vi "数据查询筛选弹框.vi"(8 "error in (no error)":errorcluster caption="错误输入（无错误）", 9 "是否初始化":enum16{"init", "keep"}(ring), 10 "database":string="database1.mdb", 11 "table":string(combo)="CODMn") -> (0 "error out":errorcluster caption="错误输出", 1 "确定输出":bool, 2 "显示项":string[](array[string]), 3 "condition":string)   [LabVIEW 2016]
uses:
  <vilib>/addons/database/Auxilliary.llb/DB Tools DataTypes.ctl
  <vilib>/picture/picture.llb/imagedata.ctl
  <vilib>/Utility/miscctls.llb/LVPointTypeDef.ctl
  <vilib>/Utility/sysdir.llb/System Directory Type.ctl
  <vilib>/addons/database/Connection.llb/DB Tools Open Connec (String).vi
  <vilib>/addons/database/Connection.llb/Conn Execute.vi
  <vilib>/addons/database/Recordset.llb/Rec Fetch Recordset Data (R).vi
  <vilib>/addons/database/Recordset.llb/Rec Destroy - Connection.vi
  <userlib>/_OpenG.lib/array/array.llb/Remove Duplicates from 1D Array (String)__ogtk.vi
  <vilib>/addons/database/_DB Variant To Data/Database Variant To Data.xnode
  <vilib>/addons/database/NI_Database_API.lvlib
panel:
  in  "背景图像":T1
  in  "实时分钟小时数据":enum32{"实时数据", "分钟数据", "小时数据"}(radio)
  in  "确定":bool
  out "自定义2single":cluster{"起始范围":string, "截止范围":string}
  out "自定义1single":cluster{"起始范围":string, "截止范围":string}
  out "自定义2筛选条件":string[](array[string])
  out "自定义1筛选条件":string[](array[string])
  in  "标签 2":string="从：\n\n\n至："
  in  "自定义数值结束 2":dbl
  in  "自定义数值起始 2":dbl
  in  "自定义结束时间 2":timestamp(xcontrol)
  in  "自定义起始时间 2":timestamp(xcontrol)
  in  "自定义 2":T2 caption="自定义"
  in  "下拉列表":string(xcontrol)
  in  "标签":string="从：\n\n\n至："
  in  "自定义数值结束":dbl
  in  "自定义数值起始":dbl
  in  "自定义结束时间":timestamp(xcontrol)
  in  "自定义起始时间":timestamp(xcontrol)
  in  "自定义":T2
  in  "下拉列表 2":string(xcontrol)
  out "type":T3[](array[typedef])
  out "所有测量模式":string[](array[string])
  out "数组":string[](array[string])
  out "columns":string[](array[string])
  in  "测量模式":T4
  in  "退出":bool
  in  "清空":bool
  in  "时间标识输入1":timestamp(xcontrol)
  in  "时间标识输入2":timestamp(xcontrol)
  # "时间"
  # "从："
  # "至："
  # "测试模式"
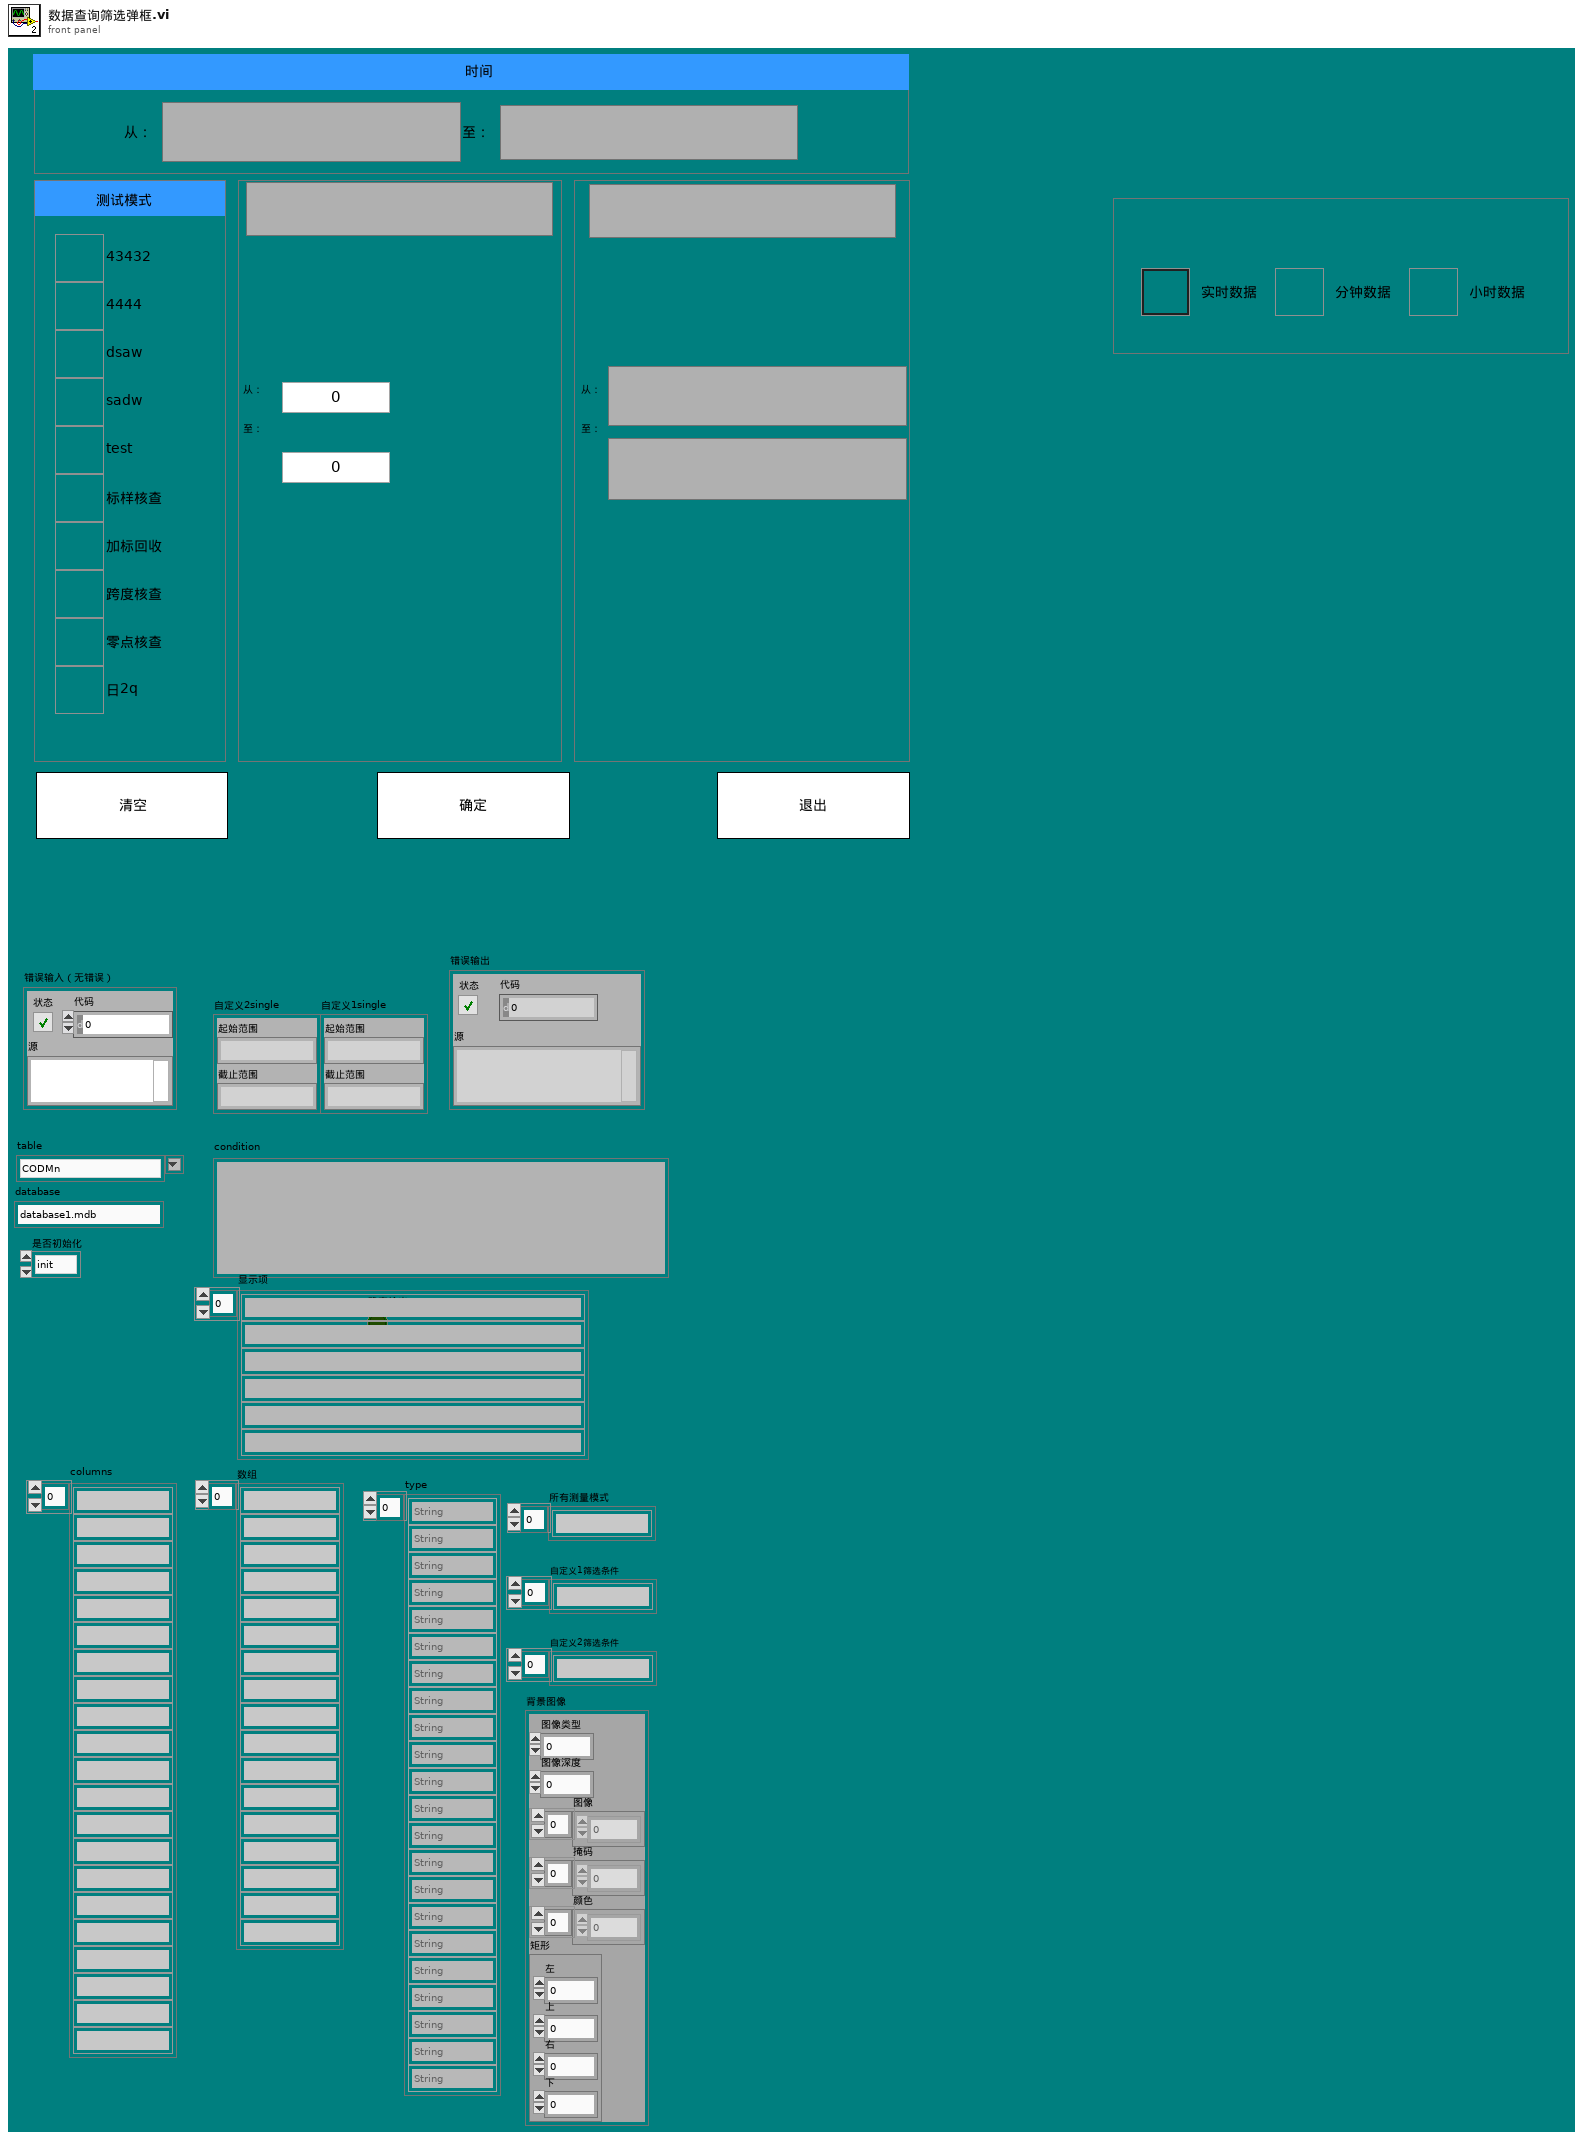
[diagram p1: front panel]
types:
  T1 = typedef "imagedata.ctl" = cluster{"image type":i32, "image depth":i32, "image":u8[], "mask":u8[], "colors":u32[], "Rectangle":cluster{"left":i16, "top":i16, "right":i16, "bottom":i16}}
  T2 = cluster{"DSADSA ":bool, "2":bool, "3":bool, "4":bool, "5":bool, "6":bool, "7":bool, "8":bool, "9":bool, "10":bool}
  T3 = typedef "NI_Database_API.lvlib/DB Tools DataTypes.ctl" = enum16{"String", "Long (I32)", "Single (SGL)", "Double (DBL)", "Date/Time", "Binary"}
  T4 = cluster{"水样测试":bool, "标样核查":bool, "零点核查":bool, "跨度核查":bool, "空白测试":bool, "平行样测试":bool, "加标回收":bool, "空白校准":bool, "标样校准":bool, "初始化清洗":bool}
  T5 = enum8{"Enabled", "Disabled", "Disabled and Grayed Out"}
  T6 = typedef "LVPointTypeDef.ctl" = cluster{"Horizontal":i16, "Vertical":i16}
  T7 = typedef "System Directory Type.ctl" = i32
  T8 = typedef "NI_Database_API.lvlib/Conn ObjectReference.ctl" = refnum<k1>
  T9 = cluster{"name":string, "database data type":T3, "defined size":i32}[]
  T10 = typedef "NI_Database_API.lvlib/Rec ObjectReference.ctl" = refnum<k1>
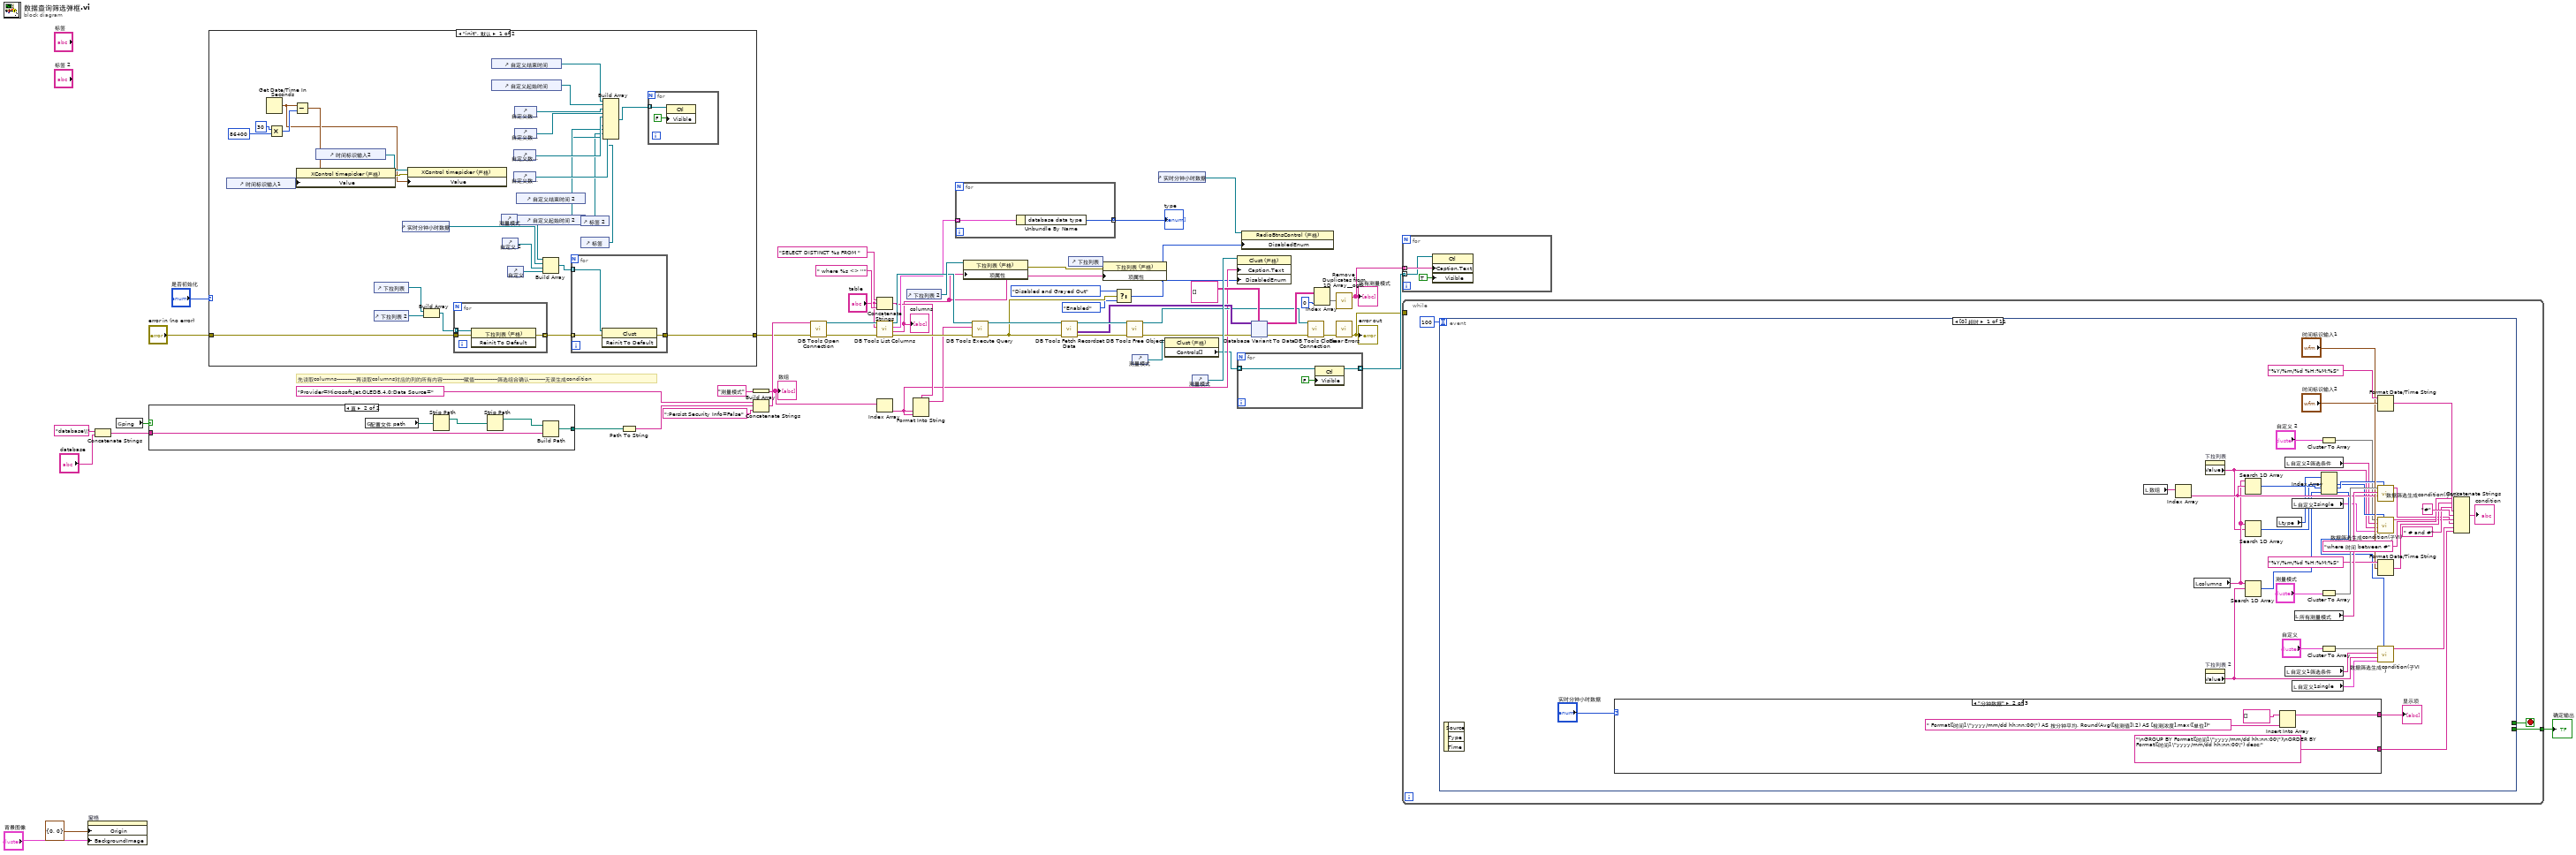
[diagram p0: block diagram]
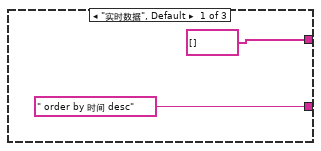
[diagram p3: hidden frame]
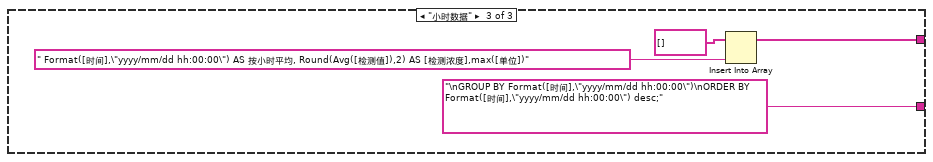
[diagram p4: hidden frame]
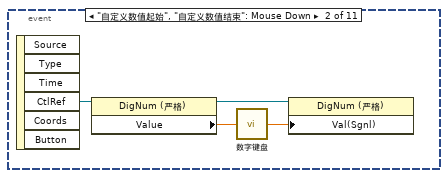
[diagram p5: hidden frame]
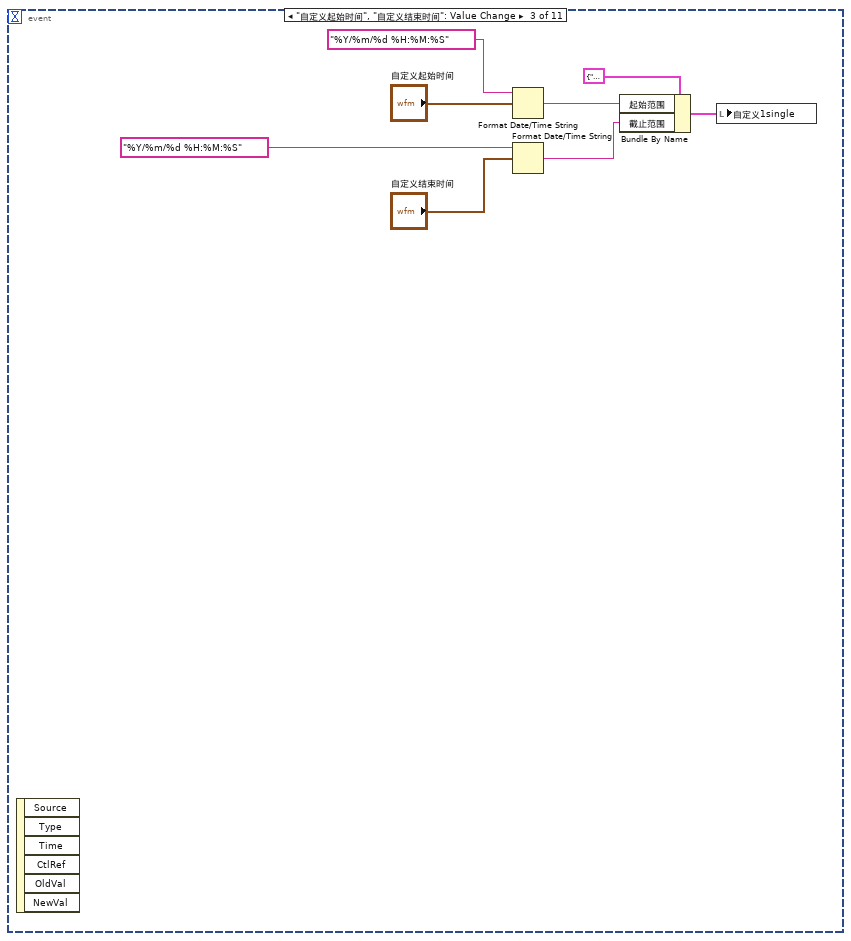
[diagram p6: hidden frame]
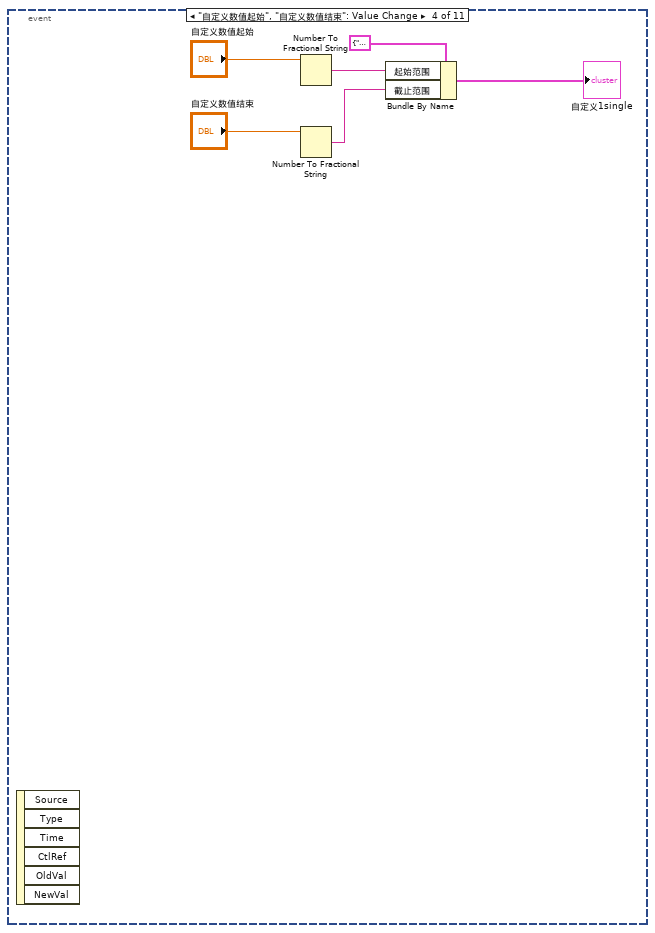
[diagram p7: hidden frame]
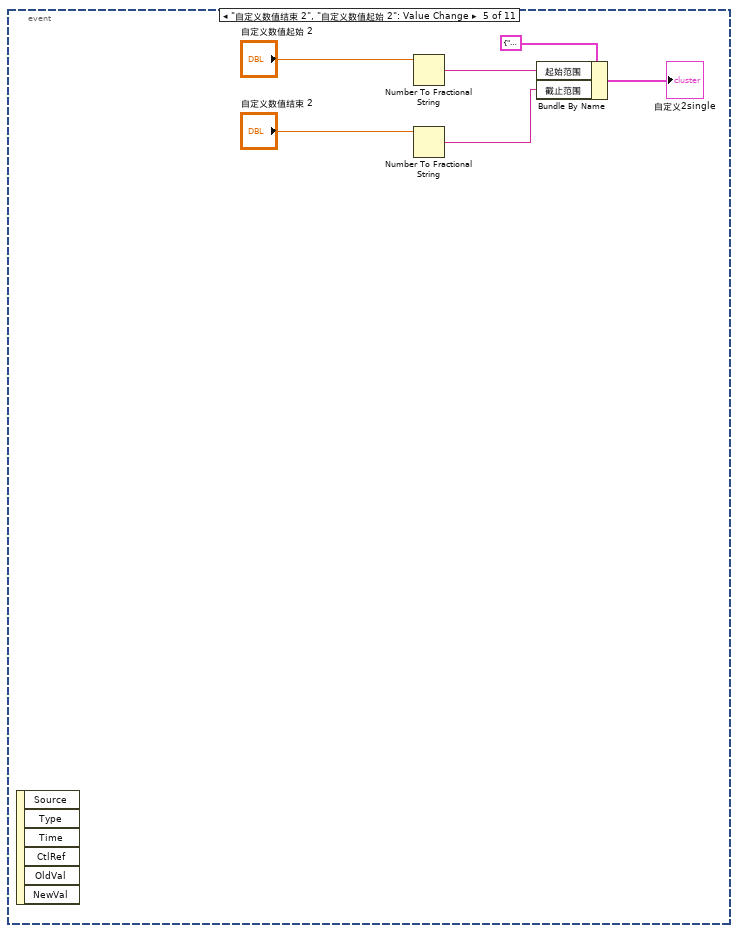
[diagram p8: hidden frame]
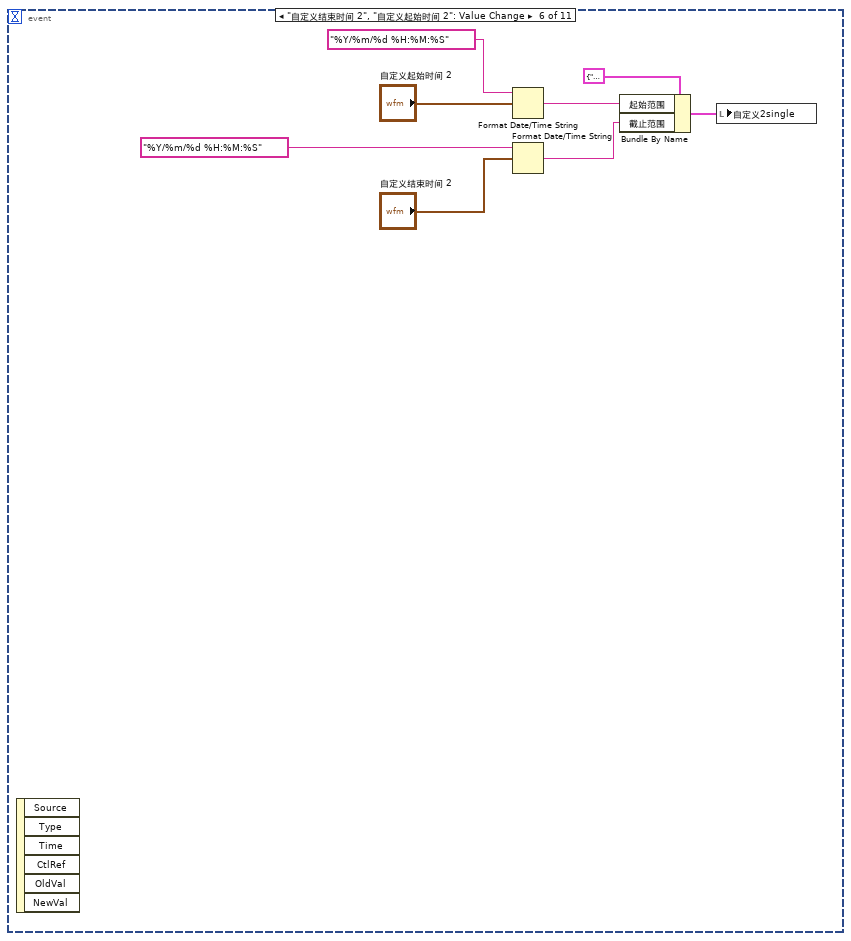
[diagram p9: hidden frame]
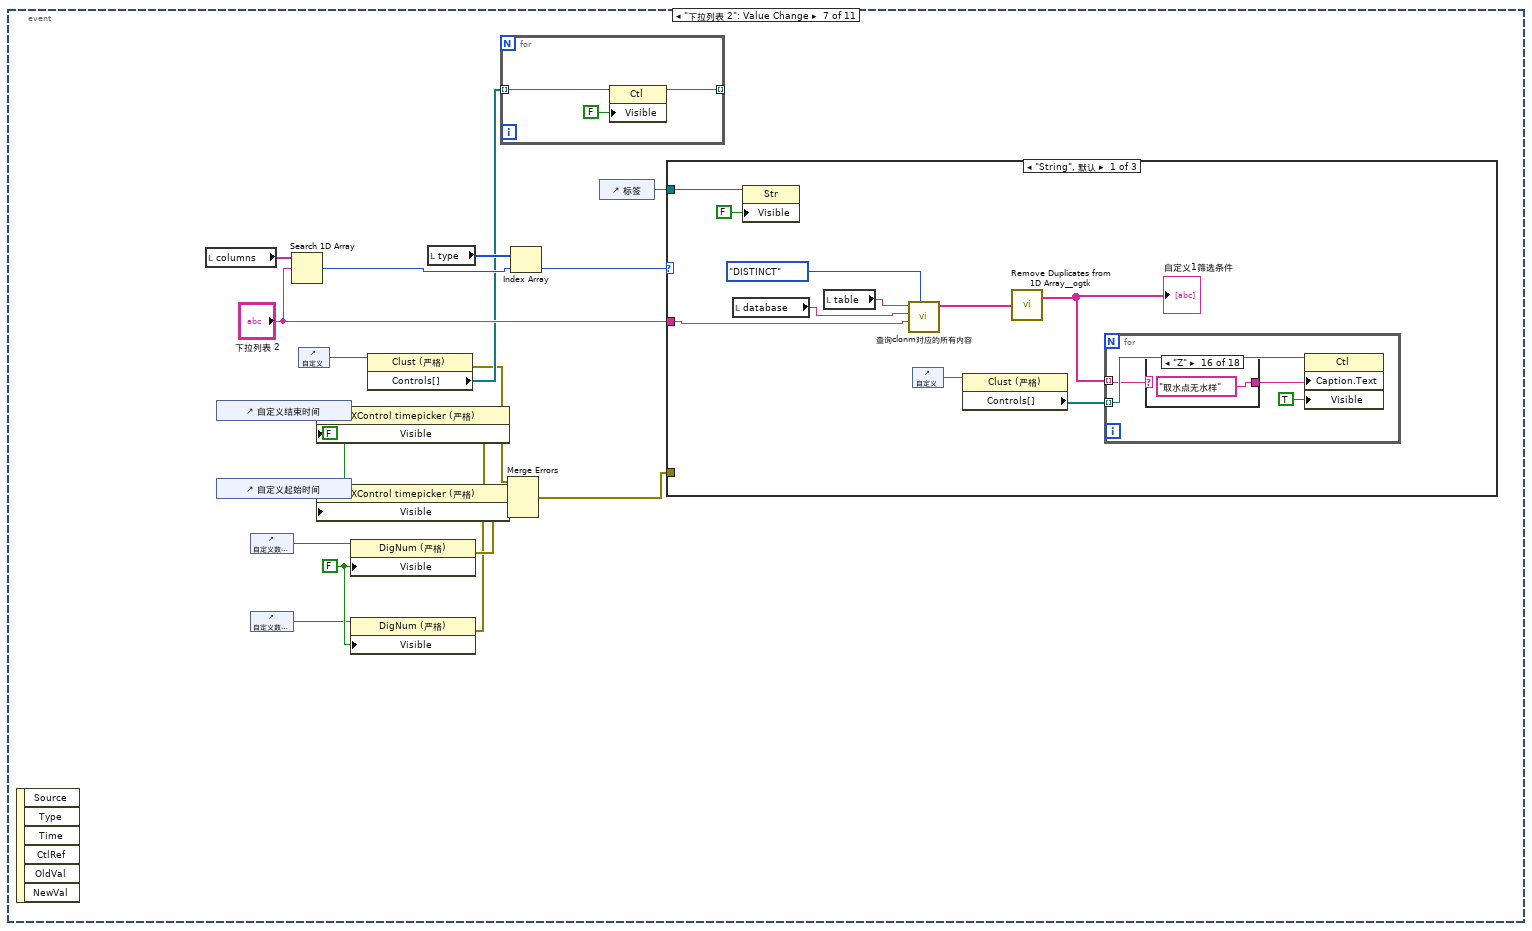
[diagram p10: hidden frame]
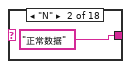
[diagram p12: hidden frame]
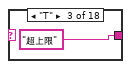
[diagram p13: hidden frame]
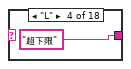
[diagram p14: hidden frame]
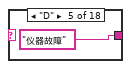
[diagram p15: hidden frame]
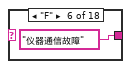
[diagram p16: hidden frame]
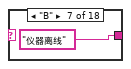
[diagram p17: hidden frame]
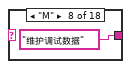
[diagram p18: hidden frame]
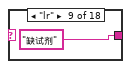
[diagram p19: hidden frame]
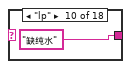
[diagram p20: hidden frame]
diagram:
  # "先读取columns-----------再读取columns对应的列的所有内容------------赋值-------------筛选组合确认---------无误生成condition"
  n1 = property on="窗格" class="Pane"("Origin"=T6 {"Horizontal"=0, "Vertical"=0} ("原点"), "BackgroundImage"="背景图像") -> ()  [unwired: 2 in, 2 out]
  n2 = Concatenate Strings("database\\" ("名称或相对路径"), "database") -> (w48:string)
  n3 = global read "ping全局.vi" "ping"() -> (w49:bool)
  n4 = case shown="真" w49 {
    tunnel: w48 -> [w58 w64]
    tunnel: [w57 w62] -> w47
    frame False {
      w59 = T7 2 items=["用户目录"=0, "用户桌面"=1, "用户文档"=2, "用户应用程序数据"=3, "用户设置"=4, "用户临时目录"=5, "公共文档"=6, "公共应用程序数据"=7, "公共设置"=8, "公共缓存"=13, "系统核心库"=9, "系统安装库"=10, "应用程序文件"=11, "启动盘根目录"=12] ("system directory type")
      n5 = call <vilib>:"Get System Directory.vi"("system directory type"=w59) -> ("system directory"=w60:path)  [unwired: 10 in]
      n6 = Build Path(base path=w60, name or relative path=w58) -> (appended path=w57:path)
    }
    frame True {
      n7 = global read "ping全局.vi" "配置文件 path"() -> (w61:path)
      n8 = Strip Path(path=w61) -> (stripped path=w65:path)  [unwired: 1 out]
      n9 = Strip Path(path=w65) -> (stripped path=w63:path)  [unwired: 1 out]
      n10 = Build Path(base path=w63, name or relative path=w64) -> (appended path=w62:path)
    }
  }
  n11 = case shown="\"init\", 默认" "是否初始化" {
    tunnel: "error in (no error)" -> [w71 w104]
    tunnel: [w90 w104] -> w8
    frame "init", Default {
      n12 = control-ref of="时间标识输入1"() -> (w73:refnum<vi>)
      n13 = Get Date/Time In Seconds() -> (seconds since 1Jan1904=w66:timestamp)
      n14 = Multiply(x=30, y=86400) -> (x*y=w85:i32)
      n15 = Subtract(x=w66, y=w85) -> (x-y=w89:timestamp)
      n16 = property class="XControl timepicker (严格)"(reference=w73, "Value"=w89) -> (error out=w88:errorcluster)  [unwired: 1 in, 1 out]
      n17 = control-ref of="时间标识输入2"() -> (w72:refnum<vi>)
      n18 = control-ref of="下拉列表"() -> (w69:refnum<vi>)
      n19 = control-ref of="下拉列表 2"() -> (w68:refnum<vi>)
      n20 = control-ref of="实时分钟小时数据"() -> (w95:refnum<vi>)
      n21 = property class="XControl timepicker (严格)"(reference=w72, error in=w88, "Value"=w66) -> ()  [unwired: 2 out]
      n22 = Build Array(w69, w68) -> (w67:refnum<vi>[])
      n23 = for {
        tunnel: w71 -> [w98]
        tunnel: [w97] -> w70 mode=indexing
        tunnel: w67 -> [w96] mode=indexing
        n24 = invoke class="下拉列表 (严格)" method="Reinit To Default"(reference=w96, error in=w98) -> (error out=w97:errorcluster)  [unwired: 1 in, 2 out]
      }
      n25 = control-ref of="自定义结束时间"() -> (w84:refnum<vi>)
      n26 = control-ref of="自定义起始时间"() -> (w83:refnum<vi>)
      n27 = control-ref of="测量模式"() -> (w91:refnum<vi>)
      n28 = control-ref of="自定义 2"() -> (w94:refnum<vi>)
      n29 = control-ref of="自定义"() -> (w93:refnum<vi>)
      n30 = control-ref of="自定义数值结束 2"() -> (w80:refnum<vi>)
      n31 = control-ref of="自定义数值起始 2"() -> (w79:refnum<vi>)
      n32 = control-ref of="自定义数值结束"() -> (w82:refnum<vi>)
      n33 = control-ref of="自定义数值起始"() -> (w81:refnum<vi>)
      n34 = control-ref of="自定义结束时间 2"() -> (w77:refnum<vi>)
      n35 = control-ref of="自定义起始时间 2"() -> (w78:refnum<vi>)
      n36 = Build Array(w91, w95, w94, w93) -> (w92:refnum<vi>[])
      n37 = for {
        tunnel: w92 -> [w103] mode=indexing
        tunnel: w70 -> [w102] mode=indexing
        tunnel: [w101] -> w90
        n38 = invoke class="Clust" method="Reinit To Default"(reference=w103, error in=w102) -> (error out=w101:errorcluster)  [unwired: 1 in, 2 out]
      }
      n39 = control-ref of="标签 2"() -> (w74:refnum<vi>)
      n40 = control-ref of="标签"() -> (w75:refnum<vi>)
      n41 = Build Array(w84, w83, w82, w81, w80, w79, w77, w78, w74, w75) -> (w76:refnum<vi>[])
      n42 = for {
        tunnel: w76 -> [w100] mode=indexing
        n43 = property class="Ctl"(reference=w100, "Visible"=FALSE ("可见")) -> ()  [unwired: 1 in, 2 out]
      }
    }
    frame "keep" {
    }
  }
  n44 = Path To String(path=w47) -> (string=w53:string)
  n45 = Build Array("测量模式" ("Element Data")) -> (w11:string[])
  "数组" <- w11
  n46 = Concatenate Strings("Provider=Microsoft.Jet.OLEDB.4.0;Data Source=", w53, ";Persist Security Info=False") -> (w52:string)
  n47 = call-poly <vilib>:"DB Tools Open Connection.vi"("error in (no error)"=w8, "connection information"=w52) -> ("error out"=w45:errorcluster, "connection reference"=w46:T8)  [unwired: 6 in]
  n48 = Concatenate Strings("SELECT DISTINCT %s FROM " ("字符串"), "table", " where %s <> ''" ("字符串")) -> (w22:string)
  n49 = call <vilib>:"DB Tools List Columns.vi"("error in (no error)"=w45, "table"="table", "connection reference"=w46) -> ("error out"=w39:errorcluster, "columns"=w1:string[], "column information"=w26:T9, "connection reference out"=w27:T8)  [unwired: 1 in]
  "columns" <- w1
  n50 = Index Array(array=w11) -> (element=w20:string)  [unwired: 1 in]
  n51 = control-ref of="下拉列表 2"() -> (w28:refnum<vi>)
  n52 = Format Into String(format string=w22, w20, w20) -> (resulting string=w38:string)  [unwired: 2 in, 1 out]
  n53 = for {
    tunnel: w26 -> [w106] mode=indexing
    tunnel: [w105] -> w25 mode=indexing
    n54 = Unbundle By Name(w106) -> ("database data type"=w105:T3)
  }
  "type" <- w25
  n55 = property class="下拉列表 (严格)"(reference=w28, "项属性"=w1) -> (error out=w7:errorcluster)  [unwired: 1 in, 1 out]
  n56 = call-poly <vilib>:"DB Tools Execute Query.vi"("error in (no error)"=w39, "SQL query"=w38, "connection reference"=w27) -> ("error out"=w19:errorcluster, "recordset reference"=w42:T10)  [unwired: 5 in]
  n57 = call-poly <vilib>:"DB Tools Fetch Recordset Data.vi"("error in (no error)"=w19, "recordset reference"=w42) -> ("error out"=w41:errorcluster, "recordset data"=w34:variant[][], "recordset reference out"=w40:T10)  [unwired: 3 in]
  n58 = control-ref of="下拉列表"() -> (w16:refnum<vi>)
  n59 = property class="下拉列表 (严格)"(reference=w16, error in=w7, "项属性"=w1) -> ()  [unwired: 2 out]
  n60 = Select(t=T5."Disabled and Grayed Out" ("禁用"), s=w19, f=T5."Enabled" ("禁用")) -> (s? t:f=w3:T5)
  n61 = call-poly <vilib>:"DB Tools Free Object.vi"("error in (no error)"=w41, "recordset reference"=w40) -> ("error out"=w33:errorcluster, "connection reference"=w32:T8)  [unwired: 8 in]
  n62 = control-ref of="测量模式"() -> (w56:refnum<vi>)
  n63 = control-ref of="实时分钟小时数据"() -> (w4:refnum<vi>)
  n64 = property class="Clust (严格)"(reference=w56) -> ("Controls[]"=w15:refnum<vi>[])  [unwired: 1 in, 2 out]
  n65 = control-ref of="测量模式"() -> (w43:refnum<vi>)
  n66 = property class="Clust (严格)"(reference=w43, "Caption.Text"=w20, "DisabledEnum"=w3) -> ()  [unwired: 1 in, 2 out]
  n67 = for {
    tunnel: w15 -> [w109] mode=indexing
    tunnel: [w107] -> w14 mode=indexing
    n68 = property class="Ctl"(reference=w109, "Visible"=FALSE ("可见")) -> (reference out=w107:refnum<vi>)  [unwired: 1 in, 1 out]
  }
  n69 = property class="RadioBtnsControl (严格)"(reference=w4, "DisabledEnum"=w3) -> ()  [unwired: 1 in, 2 out]
  n70 = xnode "Database Variant To Data"("database variant"=w34, "error in (no error)"=w33, "type"=string[][] []) -> ("data"=w35:string[][], "error out"=w36:errorcluster)
  n71 = call <vilib>:"DB Tools Close Connection.vi"("error in (no error)"=w36, "connection reference"=w32) -> ("error out"=w10:errorcluster)  [unwired: 5 in]
  n72 = Index Array(array=w35, index (col)=0 ("禁用的索引 (列)")) -> (element=w30:string[])  [unwired: 1 in]
  n73 = call-poly <userlib>:"Remove Duplicates from 1D Array__ogtk.vi"("Input Array"=w30) -> ("Output Array"=w13:string[])  [unwired: 1 out]
  "所有测量模式" <- w13
  n74 = call <vilib>:"Clear Errors.vi"("error in (no error)"=w10) -> ("error out"=w5:errorcluster)  [unwired: 5 in, 1 out]
  "error out" <- w5
  n75 = for {
    tunnel: w13 -> [w112] mode=indexing
    tunnel: w14 -> [w110] mode=indexing
    n76 = property class="Ctl"(reference=w110, "Caption.Text"=w112, "Visible"=TRUE ("可见")) -> ()  [unwired: 1 in, 2 out]
  }
  n77 = while {
    tunnel: [w113] -> w12
    tunnel: w5 -> [_]
    stop <- w115 stop-if-true
    n78 = event shown="[0] 超时" {
      selector: _ -> [_ _ _ _ _ _ _ _ _ _ _]
      dyn-events: _ -> [_ _ _ _ _ _ _ _ _ _ _]
      timeout: 100 -> [_ _ _ _ _ _ _ _ _ _ _]
      tunnel: [_ _ _ _ _ _ _ _ _ w395 TRUE] -> w115
      tunnel: [_ _ _ _ _ _ _ _ _ w395 _] -> w113
      event Timeout {
        n79 = event-data() -> ()  [unwired: 1 in, 3 out]
        n80 = case shown="\"分钟数据\"" "实时分钟小时数据" {
          tunnel: [string[] [] ("显示项") w157 w161] -> w116
          tunnel: [" order by 时间 desc" ("字符串") "\nGROUP BY Format([时间],\"yyyy/mm/dd hh:nn:00\")\nORDER BY Format([时间],\"yyyy/mm/dd hh:nn:00\") desc;" ("字符串") "\nGROUP BY Format([时间],\"yyyy/mm/dd hh:00:00\")\nORDER BY Format([时间],\"yyyy/mm/dd hh:00:00\") desc;" ("字符串")] -> w117
          frame "实时数据", Default {
          }
          frame "分钟数据" {
            n81 = Insert Into Array(array=string[] [] ("显示项"), new element=" Format([时间],\"yyyy/mm/dd hh:nn:00\") AS 按分钟平均, Round(Avg([检测值]),2) AS [检测浓度],max([单位])" ("新元素/子数组")) -> (w157:string[])  [unwired: 1 in]
          }
          frame "小时数据" {
            n82 = Insert Into Array(array=string[] [] ("显示项"), new element=" Format([时间],\"yyyy/mm/dd hh:00:00\") AS 按小时平均, Round(Avg([检测值]),2) AS [检测浓度],max([单位])" ("新元素/子数组")) -> (w161:string[])  [unwired: 1 in]
          }
        }
        "显示项" <- w116
        n83 = local read "数组"() -> (w154:string[])
        n84 = Index Array(array=w154) -> (element=w140:string)  [unwired: 1 in]
        n85 = local read "columns"() -> (w134:string[])
        n86 = property on="下拉列表" class="下拉列表 (严格)"() -> ("Value"=w125:string)  [unwired: 2 in, 2 out]
        n87 = property on="下拉列表 2" class="下拉列表 (严格)"() -> ("Value"=w124:string)  [unwired: 2 in, 2 out]
        n88 = Search 1D Array(1D array=w134, element=w140) -> (index of element=w138:i32)  [unwired: 1 in]
        n89 = Search 1D Array(1D array=w134, element=w125) -> (index of element=w133:i32)  [unwired: 1 in]
        n90 = Search 1D Array(1D array=w134, element=w124) -> (index of element=w136:i32)  [unwired: 1 in]
        n91 = local read "type"() -> (w139:T3[])
        n92 = local read "自定义2筛选条件"() -> (w122:string[])
        n93 = local read "自定义1筛选条件"() -> (w123:string[])
        n94 = local read "自定义2single"() -> (w120:cluster{"起始范围":string, "截止范围":string})
        n95 = local read "自定义1single"() -> (w119:cluster{"起始范围":string, "截止范围":string})
        n96 = local read "所有测量模式"() -> (w153:string[])
        n97 = Cluster To Array(cluster="自定义 2") -> (array=w131:bool[])
        n98 = Index Array(array=w139, index #1=w133, index #2=w138, index #3=w136) -> (element #1=w132:T3, element #2=w137:T3, element #3=w135:T3)
        n99 = Cluster To Array(cluster="测量模式") -> (array=w152:bool[])
        n100 = Cluster To Array(cluster="自定义") -> (array=w121:bool[])
        n101 = Format Date/Time String(time format string (%c)="%Y/%m/%d %H:%M:%S" ("时间格式字符串(%c)"), seconds (now)="时间标识输入2") -> (date/time string=w149:string)  [unwired: 1 in]
        n102 = call "数据筛选生成condition(子VI).vi"("database data type"=w137, "段名"=w140, "筛选内容"=w153, "簇转数组"=w152) -> ("condition"=w129:string)  [unwired: 7 in]
        n103 = call "数据筛选生成condition(子VI).vi"("database data type"=w132, "Single"=w120, "段名"=w125, "筛选内容"=w122, "簇转数组"=w131) -> ("condition"=w130:string)  [unwired: 6 in]
        n104 = Format Date/Time String(time format string (%c)="%Y/%m/%d %H:%M:%S" ("时间格式字符串(%c)"), seconds (now)="时间标识输入1") -> (date/time string=w147:string)  [unwired: 1 in]
        n105 = call "数据筛选生成condition(子VI).vi"("database data type"=w135, "Single"=w119, "段名"=w124, "筛选内容"=w123, "簇转数组"=w121) -> ("condition"=w128:string)  [unwired: 6 in]
        n106 = Concatenate Strings("where 时间 between #", w147, " # and #" ("condition"), w149, "#" ("condition"), w130, w129, w128, w117) -> (→"condition":string)
      }
      event "自定义数值起始", "自定义数值结束": Mouse Down {
        n107 = event-data() -> ("CtlRef"=w168:refnum<vi>)  [unwired: 1 in, 5 out]
        n108 = property class="DigNum (严格)"(reference=w168) -> (reference out=w166:refnum<vi>, "Value"=w167:dbl)  [unwired: 1 in, 1 out]
        n109 = call "数字键盘.vi"("OldNumber"=w167) -> ("NewNumber"=w165:sgl)
        n110 = property class="DigNum (严格)"(reference=w166, "Val(Sgnl)"=w165) -> ()  [unwired: 1 in, 2 out]
      }
      event "自定义起始时间", "自定义结束时间": Value Change {
        n111 = event-data() -> ()  [unwired: 1 in, 6 out]
        n112 = Format Date/Time String(time format string (%c)="%Y/%m/%d %H:%M:%S" ("时间格式字符串(%c)"), seconds (now)="自定义起始时间") -> (date/time string=w175:string)  [unwired: 1 in]
        n113 = Format Date/Time String(time format string (%c)="%Y/%m/%d %H:%M:%S" ("时间格式字符串(%c)"), seconds (now)="自定义结束时间") -> (date/time string=w176:string)  [unwired: 1 in]
        n114 = Bundle By Name(cluster=cluster{"起始范围":string, "截止范围":string} {"起始范围"="2", "截止范围"="5"} ("Single"), "起始范围"=w175, "截止范围"=w176) -> (w169:cluster{"起始范围":string, "截止范围":string})
        n115 = local write "自定义1single"(w169) -> ()
      }
      event "自定义数值起始", "自定义数值结束": Value Change {
        n116 = event-data() -> ()  [unwired: 1 in, 6 out]
        n117 = Number To Fractional String(number="自定义数值起始") -> (F-format string=w181:string)  [unwired: 3 in]
        n118 = Number To Fractional String(number="自定义数值结束") -> (F-format string=w182:string)  [unwired: 3 in]
        n119 = Bundle By Name(cluster=cluster{"起始范围":string, "截止范围":string} {"起始范围"="2", "截止范围"="5"} ("Single"), "起始范围"=w181, "截止范围"=w182) -> (→"自定义1single":cluster{"起始范围":string, "截止范围":string})
      }
      event "自定义数值结束 2", "自定义数值起始 2": Value Change {
        n120 = event-data() -> ()  [unwired: 1 in, 6 out]
        n121 = Number To Fractional String(number="自定义数值起始 2") -> (F-format string=w185:string)  [unwired: 3 in]
        n122 = Number To Fractional String(number="自定义数值结束 2") -> (F-format string=w184:string)  [unwired: 3 in]
        n123 = Bundle By Name(cluster=cluster{"起始范围":string, "截止范围":string} {"起始范围"="2", "截止范围"="5"} ("Single"), "起始范围"=w185, "截止范围"=w184) -> (→"自定义2single":cluster{"起始范围":string, "截止范围":string})
      }
      event "自定义结束时间 2", "自定义起始时间 2": Value Change {
        n124 = event-data() -> ()  [unwired: 1 in, 6 out]
        n125 = Format Date/Time String(time format string (%c)="%Y/%m/%d %H:%M:%S" ("时间格式字符串(%c)"), seconds (now)="自定义起始时间 2") -> (date/time string=w194:string)  [unwired: 1 in]
        n126 = Format Date/Time String(time format string (%c)="%Y/%m/%d %H:%M:%S" ("时间格式字符串(%c)"), seconds (now)="自定义结束时间 2") -> (date/time string=w195:string)  [unwired: 1 in]
        n127 = Bundle By Name(cluster=cluster{"起始范围":string, "截止范围":string} {"起始范围"="2", "截止范围"="5"} ("Single"), "起始范围"=w194, "截止范围"=w195) -> (w196:cluster{"起始范围":string, "截止范围":string})
        n128 = local write "自定义2single"(w196) -> ()
      }
      event "下拉列表 2": Value Change {
        w207 = FALSE ("可见")
        w197 = FALSE ("可见")
        n129 = event-data() -> ()  [unwired: 1 in, 6 out]
        n130 = local read "columns"() -> (w214:string[])
        n131 = control-ref of="自定义结束时间"() -> (w209:refnum<vi>)
        n132 = control-ref of="自定义起始时间"() -> (w208:refnum<vi>)
        n133 = control-ref of="自定义数值结束"() -> (w206:refnum<vi>)
        n134 = control-ref of="自定义数值起始"() -> (w199:refnum<vi>)
        n135 = Search 1D Array(1D array=w214, element="下拉列表 2") -> (index of element=w216:i32)  [unwired: 1 in]
        n136 = control-ref of="自定义"() -> (w211:refnum<vi>)
        n137 = property class="XControl timepicker (严格)"(reference=w209, "Visible"=w197) -> (error out=w204:errorcluster)  [unwired: 1 in, 1 out]
        n138 = property class="XControl timepicker (严格)"(reference=w208, "Visible"=w197) -> (error out=w203:errorcluster)  [unwired: 1 in, 1 out]
        n139 = property class="DigNum (严格)"(reference=w206, "Visible"=w207) -> (error out=w202:errorcluster)  [unwired: 1 in, 1 out]
        n140 = property class="DigNum (严格)"(reference=w199, "Visible"=w207) -> (error out=w201:errorcluster)  [unwired: 1 in, 1 out]
        n141 = property class="Clust (严格)"(reference=w211) -> (error out=w205:errorcluster, "Controls[]"=w210:refnum<vi>[])  [unwired: 1 in, 1 out]
        n142 = local read "type"() -> (w215:T3[])
        n143 = for {
          tunnel: w210 -> [w219] mode=indexing
          tunnel: [w217] -> _ mode=indexing
          n144 = property class="Ctl"(reference=w219, "Visible"=FALSE ("可见")) -> (reference out=w217:refnum<vi>)  [unwired: 1 in, 1 out]
        }
        n145 = Merge Errors(w205, w204, w203, w202, w201) -> (w200:errorcluster)
        n146 = Index Array(array=w215, index=w216) -> (element=w212:T3)
        n147 = control-ref of="标签"() -> (w198:refnum<vi>)
        n148 = case shown="\"String\", 默认" w212 {
          tunnel: "下拉列表 2" -> [w227 w259 w280]
          tunnel: w200 -> [_ _ _]
          tunnel: w198 -> [w222 w265 w285]
          frame "String", Default {
            n149 = local read "database"() -> (w228:string)
            n150 = property class="Str"(reference=w222, "Visible"=FALSE ("可见")) -> ()  [unwired: 1 in, 2 out]
            n151 = local read "table"() -> (w229:string)
            n152 = call "查询clonm对应的所有内容.vi"("条件"=enum16{"DISTINCT", "MIN", "MAX"}."DISTINCT", "组合框"=w227, "database"=w228, "table"=w229) -> ("输出数组"=w226:string[])  [unwired: 6 in, 1 out]
            n153 = control-ref of="自定义"() -> (w224:refnum<vi>)
            n154 = property class="Clust (严格)"(reference=w224) -> ("Controls[]"=w223:refnum<vi>[])  [unwired: 1 in, 2 out]
            n155 = call-poly <userlib>:"Remove Duplicates from 1D Array__ogtk.vi"("Input Array"=w226) -> ("Output Array"=w225:string[])  [unwired: 1 out]
            "自定义1筛选条件" <- w225
            n156 = for {
              tunnel: w225 -> [w230] mode=indexing
              tunnel: w223 -> [w232] mode=indexing
              n157 = case shown="\"Z\"" w230 {
                selector: w230 -> [w234 _ _ _ _ _ _ _ _ _ _ _ _ _ _ _ _ _]
                tunnel: [w234 "正常数据" "超上限" "超下限" "仪器故障" "仪器通信故障" "仪器离线" "维护调试数据" "缺试剂" "缺纯水" "缺水样" "缺标液" "加标回收" "平行样测试" "电源故障" "取水点无水样" "手工输入数据" "手动测试数据"] -> w231
                frame Default {
                }
                frame "N" {
                }
                frame "T" {
                }
                frame "L" {
                }
                frame "D" {
                }
                frame "F" {
                }
                frame "B" {
                }
                frame "M" {
                }
                frame "lr" {
                }
                frame "lp" {
                }
                frame "lw" {
                }
                frame "ls" {
                }
                frame "ra" {
                }
                frame "pt" {
                }
                frame "P" {
                }
                frame "Z" {
                }
                frame "S" {
                }
                frame "hd" {
                }
              }
              n158 = property class="Ctl"(reference=w232, "Caption.Text"=w231, "Visible"=TRUE ("可见")) -> ()  [unwired: 1 in, 2 out]
            }
          }
          frame "Long (I32)".."Double (DBL)" {
            w267 = TRUE ("可见")
            n159 = local read "database"() -> (w260:string)
            n160 = property class="Str"(reference=w265, "Visible"=TRUE ("可见")) -> ()  [unwired: 1 in, 2 out]
            n161 = local read "table"() -> (w261:string)
            n162 = call "查询clonm对应的所有内容.vi"("条件"=enum16{"DISTINCT", "MIN", "MAX"}."MAX", "组合框"=w259, "database"=w260, "table"=w261) -> ("输出数组"=w258:string[])  [unwired: 6 in, 1 out]
            n163 = call "查询clonm对应的所有内容.vi"("条件"=enum16{"DISTINCT", "MIN", "MAX"}."MIN", "组合框"=w259, "database"=w260, "table"=w261) -> ("输出数组"=w263:string[])  [unwired: 6 in, 1 out]
            n164 = Index Array(array=w258) -> (element=w253:string)  [unwired: 1 in]
            n165 = Index Array(array=w263) -> (element=w252:string)  [unwired: 1 in]
            n166 = control-ref of="自定义数值结束"() -> (w268:refnum<vi>)
            n167 = control-ref of="自定义数值起始"() -> (w269:refnum<vi>)
            n168 = Fract/Exp String To Number(string=w253) -> (number=w256:dbl)  [unwired: 3 in, 1 out]
            n169 = Fract/Exp String To Number(string=w252) -> (number=w257:dbl)  [unwired: 3 in, 1 out]
            n170 = Bundle By Name(cluster=cluster{"起始范围":string, "截止范围":string} {"起始范围"="2", "截止范围"="5"} ("Single"), "起始范围"=w252, "截止范围"=w253) -> (w254:cluster{"起始范围":string, "截止范围":string})
            n171 = property class="DigNum (严格)"(reference=w268, "Visible"=w267, "Value"=w256) -> ()  [unwired: 1 in, 2 out]
            n172 = property class="DigNum (严格)"(reference=w269, "Visible"=w267, "Value"=w257) -> ()  [unwired: 1 in, 2 out]
            n173 = local write "自定义1single"(w254) -> ()
          }
          frame "Date/Time" {
            n174 = local read "database"() -> (w281:string)
            n175 = property class="Str"(reference=w285, "Visible"=TRUE ("可见")) -> ()  [unwired: 1 in, 2 out]
            n176 = local read "table"() -> (w282:string)
            n177 = call "查询clonm对应的所有内容.vi"("条件"=enum16{"DISTINCT", "MIN", "MAX"}."MAX", "组合框"=w280, "database"=w281, "table"=w282) -> ("输出数组"=w279:string[])  [unwired: 6 in, 1 out]
            n178 = call "查询clonm对应的所有内容.vi"("条件"=enum16{"DISTINCT", "MIN", "MAX"}."MIN", "组合框"=w280, "database"=w281, "table"=w282) -> ("输出数组"=w274:string[])  [unwired: 6 in, 1 out]
            n179 = Index Array(array=w279) -> (element=w273:string)  [unwired: 1 in]
            n180 = Index Array(array=w274) -> (element=w271:string)  [unwired: 1 in]
            n181 = call "格式日期时间字符串.vi"("data[0]"=w273) -> ("日期/时间字符串"=w272:string)  [unwired: 10 in]
            n182 = call "格式日期时间字符串.vi"("data[0]"=w271) -> ("日期/时间字符串"=w270:string)  [unwired: 10 in]
            n183 = control-ref of="自定义起始时间"() -> (w287:refnum<vi>)
            n184 = control-ref of="自定义结束时间"() -> (w288:refnum<vi>)
            n185 = call "日期字符串格式至时间格式转换(子VI).vi"("data[0]"=w272) -> ("time stamp"=w277:timestamp)  [unwired: 10 in]
            n186 = call "日期字符串格式至时间格式转换(子VI).vi"("data[0]"=w270) -> ("time stamp"=w278:timestamp)  [unwired: 10 in]
            n187 = Bundle By Name(cluster=cluster{"起始范围":string, "截止范围":string} {"起始范围"="2", "截止范围"="5"} ("Single"), "起始范围"=w270, "截止范围"=w272) -> (w275:cluster{"起始范围":string, "截止范围":string})
            n188 = property class="XControl timepicker (严格)"(reference=w287, "Visible"=TRUE ("可见"), "Value"=w278) -> ()  [unwired: 1 in, 2 out]
            n189 = property class="XControl timepicker (严格)"(reference=w288, "Visible"=TRUE ("可见"), "Value"=w277) -> ()  [unwired: 1 in, 2 out]
            n190 = local write "自定义1single"(w275) -> ()
          }
        }
      }
      event "下拉列表": Value Change {
        w301 = FALSE ("可见")
        w291 = FALSE ("可见")
        n191 = event-data() -> ()  [unwired: 1 in, 6 out]
        n192 = local read "columns"() -> (w307:string[])
        n193 = control-ref of="自定义结束时间 2"() -> (w303:refnum<vi>)
        n194 = control-ref of="自定义起始时间 2"() -> (w302:refnum<vi>)
        n195 = control-ref of="自定义数值结束 2"() -> (w300:refnum<vi>)
        n196 = control-ref of="自定义数值起始 2"() -> (w293:refnum<vi>)
        n197 = control-ref of="自定义 2"() -> (w305:refnum<vi>)
        n198 = Search 1D Array(1D array=w307, element="下拉列表") -> (index of element=w309:i32)  [unwired: 1 in]
        n199 = property class="XControl timepicker (严格)"(reference=w303, "Visible"=w291) -> (error out=w298:errorcluster)  [unwired: 1 in, 1 out]
        n200 = property class="XControl timepicker (严格)"(reference=w302, "Visible"=w291) -> (error out=w297:errorcluster)  [unwired: 1 in, 1 out]
        n201 = property class="DigNum (严格)"(reference=w300, "Visible"=w301) -> (error out=w296:errorcluster)  [unwired: 1 in, 1 out]
        n202 = property class="DigNum (严格)"(reference=w293, "Visible"=w301) -> (error out=w295:errorcluster)  [unwired: 1 in, 1 out]
        n203 = property class="Clust (严格)"(reference=w305) -> (error out=w299:errorcluster, "Controls[]"=w304:refnum<vi>[])  [unwired: 1 in, 1 out]
        n204 = local read "type"() -> (w308:T3[])
        n205 = for {
          tunnel: w304 -> [w313] mode=indexing
          tunnel: [w311] -> _ mode=indexing
          n206 = property class="Ctl"(reference=w313, "Visible"=FALSE ("可见")) -> (reference out=w311:refnum<vi>)  [unwired: 1 in, 1 out]
        }
        n207 = Merge Errors(w299, w298, w297, w296, w295) -> (w294:errorcluster)
        n208 = Index Array(array=w308, index=w309) -> (element=w306:T3)
        n209 = control-ref of="标签 2"() -> (w292:refnum<vi>)
        n210 = case shown="\"String\", 默认" w306 {
          tunnel: "下拉列表" -> [w321 w354 w372]
          tunnel: w294 -> [_ _ _]
          tunnel: w292 -> [w317 w359 w379]
          frame "String", Default {
            n211 = local read "database"() -> (w322:string)
            n212 = property class="Str"(reference=w317, "Visible"=FALSE ("可见")) -> ()  [unwired: 1 in, 2 out]
            n213 = local read "table"() -> (w323:string)
            n214 = control-ref of="自定义 2"() -> (w319:refnum<vi>)
            n215 = call "查询clonm对应的所有内容.vi"("条件"=enum16{"DISTINCT", "MIN", "MAX"}."DISTINCT", "组合框"=w321, "database"=w322, "table"=w323) -> ("输出数组"=w320:string[])  [unwired: 6 in, 1 out]
            n216 = property class="Clust (严格)"(reference=w319) -> ("Controls[]"=w318:refnum<vi>[])  [unwired: 1 in, 2 out]
            n217 = call-poly <userlib>:"Remove Duplicates from 1D Array__ogtk.vi"("Input Array"=w320) -> ("Output Array"=w314:string[])  [unwired: 1 out]
            "自定义2筛选条件" <- w314
            n218 = for {
              tunnel: w314 -> [w325] mode=indexing
              tunnel: w318 -> [w326] mode=indexing
              n219 = case shown="\"Z\"" w325 {
                selector: w325 -> [w328 _ _ _ _ _ _ _ _ _ _ _ _ _ _ _ _ _]
                tunnel: [w328 "正常数据" "超上限" "超下限" "仪器故障" "仪器通信故障" "仪器离线" "维护调试数据" "缺试剂" "缺纯水" "缺水样" "缺标液" "加标回收" "平行样测试" "电源故障" "取水点无水样" "手工输入数据" "手动测试数据"] -> w324
                frame Default {
                }
                frame "N" {
                }
                frame "T" {
                }
                frame "L" {
                }
                frame "D" {
                }
                frame "F" {
                }
                frame "B" {
                }
                frame "M" {
                }
                frame "lr" {
                }
                frame "lp" {
                }
                frame "lw" {
                }
                frame "ls" {
                }
                frame "ra" {
                }
                frame "pt" {
                }
                frame "P" {
                }
                frame "Z" {
                }
                frame "S" {
                }
                frame "hd" {
                }
              }
              n220 = property class="Ctl"(reference=w326, "Caption.Text"=w324, "Visible"=TRUE ("可见")) -> ()  [unwired: 1 in, 2 out]
            }
          }
          frame "Long (I32)".."Double (DBL)" {
            w361 = TRUE ("可见")
            n221 = local read "database"() -> (w355:string)
            n222 = property class="Str"(reference=w359, "Visible"=TRUE ("可见")) -> ()  [unwired: 1 in, 2 out]
            n223 = local read "table"() -> (w356:string)
            n224 = call "查询clonm对应的所有内容.vi"("条件"=enum16{"DISTINCT", "MIN", "MAX"}."MAX", "组合框"=w354, "database"=w355, "table"=w356) -> ("输出数组"=w353:string[])  [unwired: 6 in, 1 out]
            n225 = call "查询clonm对应的所有内容.vi"("条件"=enum16{"DISTINCT", "MIN", "MAX"}."MIN", "组合框"=w354, "database"=w355, "table"=w356) -> ("输出数组"=w348:string[])  [unwired: 6 in, 1 out]
            n226 = Index Array(array=w353) -> (element=w346:string)  [unwired: 1 in]
            n227 = Index Array(array=w348) -> (element=w347:string)  [unwired: 1 in]
            n228 = control-ref of="自定义数值结束 2"() -> (w362:refnum<vi>)
            n229 = control-ref of="自定义数值起始 2"() -> (w363:refnum<vi>)
            n230 = Fract/Exp String To Number(string=w346) -> (number=w351:dbl)  [unwired: 3 in, 1 out]
            n231 = Fract/Exp String To Number(string=w347) -> (number=w352:dbl)  [unwired: 3 in, 1 out]
            n232 = Bundle By Name(cluster=cluster{"起始范围":string, "截止范围":string} {"起始范围"="2", "截止范围"="5"} ("Single"), "起始范围"=w347, "截止范围"=w346) -> (w350:cluster{"起始范围":string, "截止范围":string})
            n233 = property class="DigNum (严格)"(reference=w362, "Visible"=w361, "Value"=w351) -> ()  [unwired: 1 in, 2 out]
            n234 = property class="DigNum (严格)"(reference=w363, "Visible"=w361, "Value"=w352) -> ()  [unwired: 1 in, 2 out]
            n235 = local write "自定义2single"(w350) -> ()
          }
          frame "Date/Time" {
            n236 = local read "database"() -> (w375:string)
            n237 = property class="Str"(reference=w379, "Visible"=TRUE ("可见")) -> ()  [unwired: 1 in, 2 out]
            n238 = local read "table"() -> (w376:string)
            n239 = call "查询clonm对应的所有内容.vi"("条件"=enum16{"DISTINCT", "MIN", "MAX"}."MAX", "组合框"=w372, "database"=w375, "table"=w376) -> ("输出数组"=w374:string[])  [unwired: 6 in, 1 out]
            n240 = call "查询clonm对应的所有内容.vi"("条件"=enum16{"DISTINCT", "MIN", "MAX"}."MIN", "组合框"=w372, "database"=w375, "table"=w376) -> ("输出数组"=w373:string[])  [unwired: 6 in, 1 out]
            n241 = Index Array(array=w374) -> (element=w367:string)  [unwired: 1 in]
            n242 = Index Array(array=w373) -> (element=w365:string)  [unwired: 1 in]
            n243 = call "格式日期时间字符串.vi"("data[0]"=w367) -> ("日期/时间字符串"=w366:string)  [unwired: 10 in]
            n244 = call "格式日期时间字符串.vi"("data[0]"=w365) -> ("日期/时间字符串"=w364:string)  [unwired: 10 in]
            n245 = control-ref of="自定义起始时间 2"() -> (w381:refnum<vi>)
            n246 = control-ref of="自定义结束时间 2"() -> (w382:refnum<vi>)
            n247 = call "日期字符串格式至时间格式转换(子VI).vi"("data[0]"=w366) -> ("time stamp"=w371:timestamp)  [unwired: 10 in]
            n248 = call "日期字符串格式至时间格式转换(子VI).vi"("data[0]"=w364) -> ("time stamp"=w370:timestamp)  [unwired: 10 in]
            n249 = Bundle By Name(cluster=cluster{"起始范围":string, "截止范围":string} {"起始范围"="2", "截止范围"="5"} ("Single"), "起始范围"=w364, "截止范围"=w366) -> (w369:cluster{"起始范围":string, "截止范围":string})
            n250 = property class="XControl timepicker (严格)"(reference=w382, "Visible"=TRUE ("可见"), "Value"=w371) -> ()  [unwired: 1 in, 2 out]
            n251 = property class="XControl timepicker (严格)"(reference=w381, "Visible"=TRUE ("可见"), "Value"=w370) -> ()  [unwired: 1 in, 2 out]
            n252 = local write "自定义2single"(w369) -> ()
          }
        }
      }
      event "清空": Value Change {
        n253 = event-data() -> ()  [unwired: 1 in, 6 out]
        n254 = control-ref of="实时分钟小时数据"() -> (w388:refnum<vi>)
        n255 = control-ref of="下拉列表"() -> (w387:refnum<vi>)
        n256 = control-ref of="下拉列表 2"() -> (w386:refnum<vi>)
        n257 = control-ref of="测量模式"() -> (w392:refnum<vi>)
        n258 = control-ref of="自定义 2"() -> (w389:refnum<vi>)
        n259 = control-ref of="自定义"() -> (w390:refnum<vi>)
        n260 = Build Array(w387, w386) -> (w385:refnum<vi>[])
        n261 = Build Array(w392, w388, w389, w390) -> (w391:refnum<vi>[])
        n262 = for {
          tunnel: w385 -> [w393] mode=indexing
          n263 = invoke class="下拉列表 (严格)" method="Reinit To Default"(reference=w393) -> ()  [unwired: 2 in, 3 out]
        }
        n264 = for {
          tunnel: w391 -> [w394] mode=indexing
          n265 = invoke class="Clust" method="Reinit To Default"(reference=w394) -> ()  [unwired: 2 in, 3 out]
        }
      }
      event "确定": Value Change {
        w395 = TRUE
        n266 = event-data() -> ()  [unwired: 1 in, 6 out]
      }
      event "退出": Value Change {
        n267 = event-data() -> ()  [unwired: 1 in, 6 out]
      }
    }
  }
  "确定输出" <- w12
